vi "decrease_motor_pow.vi"(0 "delay_per_step":u32, 1 "min_pow":i32) -> ()   [LabVIEW 2017]
uses:
  Untitled Project 6/GlobalVar.vi
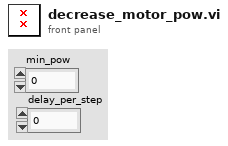
[diagram p1: front panel]
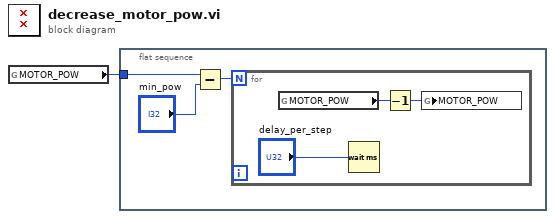
[diagram p0: block diagram]
diagram:
  n1 = global read "GlobalVar.vi" "MOTOR_POW"() -> (w1:i8)
  n2 = flat-sequence {
    tunnel: w1 -> [w4]
    frame #0 {
      n3 = Subtract(x=w4, y="min_pow") -> (x-y=w2:i32)
      n4 = for {
        N: w2 -> [_]
        n5 = global read "GlobalVar.vi" "MOTOR_POW"() -> (w6:i8)
        n6 = Wait (ms)(milliseconds to wait="delay_per_step") -> ()  [unwired: 1 out]
        n7 = Decrement(x=w6) -> (x-1=w5:i8)
        n8 = global write "GlobalVar.vi" "MOTOR_POW"(w5) -> ()
      }
    }
  }
